vi "Teleop.vi"   [LabVIEW 2016]
doc: "This VI is called for each TeleOp packet received from the DS where the robot is not disabled. It is often used to read from the joysticks and update I/O or to update setpoints for timed control loops. It should complete and return within 20 milliseconds or it may miss DS packets."
uses:
  <vilib>/Rock Robotics/WPI/Utilities/WPI_GetSetVariantRefNum.vi
  External/2ndContollerStatus.vi
  External/External.lvlib
types:
  T1 = enum16{"A", "B", "X", "Y", "LB", "RB", "Back", "Start", "Left Joystick Pressure Button", "Right Joystick Pressure Button"}
  T2 = enum16{"Left X Axis", "Left Y Axis", "Left Trigger", "Right Trigger", "Right X Axis", "Right Y Axis"}
  T3 = enum16{"A", "B", "X", "Y", "LB", "RB", "Back", "Start"}
  T4 = typedef "WPI_JoystickDevRef.ctl" = cluster{"Device":T5}
  T5 = typedef "WPI_JoystickDeviceEnum.ctl" = enum16{"USB 0", "USB 1", "USB 2", "USB 3", "USB 4", "USB 5"}
  T6 = typedef "WPI_RobotDriveDevRef.ctl" = cluster{"DevStatus":errorcluster, "Motors[]":T7[], "Square Inputs":bool, "Max Output":dbl}
  T7 = typedef "WPI_MotorControlDeviceRef.ctl" = cluster{"DeviceStatus":errorcluster, "Type":T8, "PWM":cluster{"PWM Channel":T9, "DeadBand":T10}, "CAN":cluster{"Device Number":u8, "SetOutput VI Ref":variant, "GetOutput VI Ref":variant, "Enable VI Ref":variant, "Disable VI Ref":variant, "Data":variant}, "Invert":bool}
  T8 = typedef "WPI_MotorControlType.ctl" = enum16{"PWM", "CAN"}
  T9 = typedef "FPGA_DIOPWMChannel.ctl" = enum8{"PWM 0", "PWM 1", "PWM 2", "PWM 3", "PWM 4", "PWM 5", "PWM 6", "PWM 7", "PWM 8", "PWM 9", "PWM MXP 0", "PWM MXP 1", "PWM MXP 2", "PWM MXP 3", "PWM MXP 4", "PWM MXP 5", "PWM MXP 6", "PWM MXP 7", "PWM MXP 8", "PWM MXP 9", "Invalid"}
  T10 = typedef "WPI_PWMDeadband.ctl" = cluster{"Name":string, "maxPositivePwm":i32, "minPositivePwm":i32, "centerPwm":i32, "maxNegativePwm":i32, "minNegativePwm":i32, "angularRange":u16}
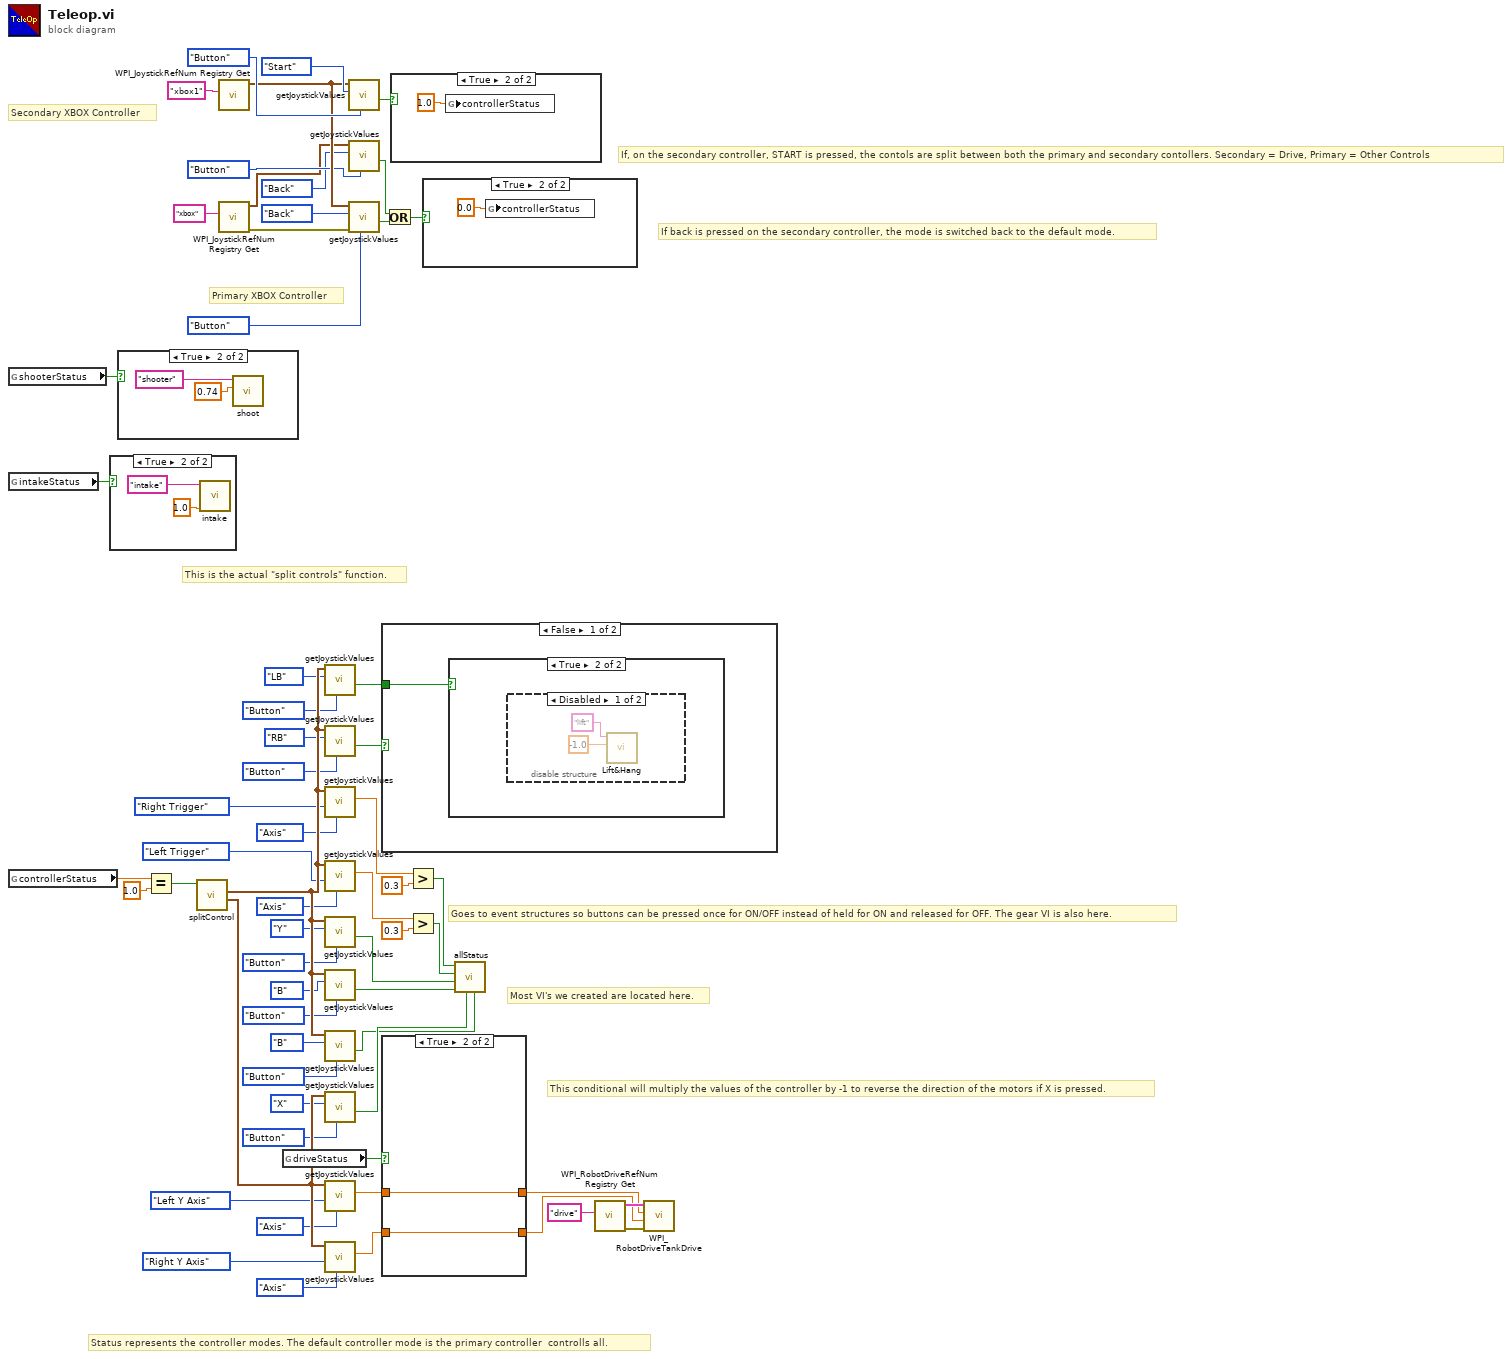
[diagram p0: block diagram]
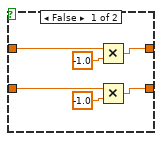
[diagram p2: hidden frame]
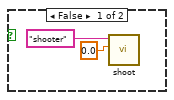
[diagram p3: hidden frame]
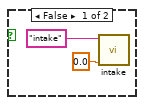
[diagram p4: hidden frame]
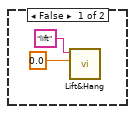
[diagram p5: hidden frame]
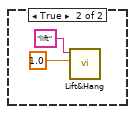
[diagram p7: hidden frame]
diagram:
  # "This is the actual \"split controls\" function."
  # "Most VI's we created are located here."
  # "This conditional will multiply the values of the controller by -1 to reverse the direction of the motors if X is pressed."
  # "Goes to event structures so buttons can be pressed once for ON/OFF instead of held for ON and released for OFF. The gear VI is also here."
  # "Status represents the controller modes. The default controller mode is the primary controller  controlls all."
  # "Secondary XBOX Controller"
  # "Primary XBOX Controller"
  # "If back is pressed on the secondary controller, the mode is switched back to the default mode."
  # "If, on the secondary controller, START is pressed, the contols are split between both the primary and secondary contollers. Secondary = Drive, Primary = Other Controls"
  n1 = global read "2ndContollerStatus.vi" "shooterStatus"() -> (w35:bool)
  n2 = global read "2ndContollerStatus.vi" "intakeStatus"() -> (w36:bool)
  n3 = global read "2ndContollerStatus.vi" "controllerStatus"() -> (w38:dbl)
  n4 = case shown="True" w36 {
    frame False {
      n5 = call "intake.vi"("intakeSpeed"=0.0, "intake"="intake") -> ()  [unwired: 9 in, 1 out]
    }
    frame True {
      n6 = call "intake.vi"("intakeSpeed"=1.0, "intake"="intake") -> ()  [unwired: 9 in, 1 out]
    }
  }
  n7 = case shown="True" w35 {
    frame False {
      n8 = call "shoot.vi"("Motor Power"=0.0, "refnum name"="shooter") -> ()  [unwired: 9 in, 1 out]
    }
    frame True {
      n9 = call "shoot.vi"("Motor Power"=0.74, "refnum name"="shooter") -> ()  [unwired: 9 in, 1 out]
    }
  }
  n10 = Equal?(x=w38, y=1.0) -> (x = y?=w24:bool)
  n11 = call "splitControl.vi"("driveStatus"=w24) -> ("JoystickDevRef 2"=w22:T4, "JoystickDevRef"=w23:T4)  [unwired: 9 in]
  n12 = call <vilib>:"WPI_JoystickRefNum Registry Get.vi"("refnum name"="xbox1" ("xbox1")) -> ("JoystickDevRef"=w57:T4)  [unwired: 9 in, 1 out]
  n13 = call <vilib>:"WPI_JoystickRefNum Registry Get.vi"("refnum name"="xbox" ("xbox")) -> ("error out"=w56:errorcluster, "JoystickDevRef"=w49:T4)  [unwired: 9 in]
  n14 = global read "2ndContollerStatus.vi" "driveStatus"() -> (w30:bool)
  n15 = call "getJoystickValues.vi"("Mode"=enum16{"Axis", "Button", "POV"}."Button", "buttonType"=T1."LB", "JoystickDevRef"=w23) -> ("Button Pressed"=w46:bool)  [unwired: 5 in, 3 out]
  n16 = call "getJoystickValues.vi"("Mode"=enum16{"Axis", "Button", "POV"}."Button", "buttonType"=T1."RB", "JoystickDevRef"=w23) -> ("Button Pressed"=w47:bool)  [unwired: 5 in, 3 out]
  n17 = call "getJoystickValues.vi"("Mode"=enum16{"Axis", "Button", "POV"}."Axis", "axisType"=T2."Right Trigger", "JoystickDevRef"=w23) -> ("Value"=w40:dbl)  [unwired: 5 in, 3 out]
  n18 = call "getJoystickValues.vi"("Mode"=enum16{"Axis", "Button", "POV"}."Axis", "axisType"=T2."Left Trigger", "JoystickDevRef"=w23) -> ("Value"=w39:dbl)  [unwired: 5 in, 3 out]
  n19 = call "getJoystickValues.vi"("Mode"=enum16{"Axis", "Button", "POV"}."Button", "buttonType"=T1."Y", "JoystickDevRef"=w23) -> ("Button Pressed"=w21:bool)  [unwired: 5 in, 3 out]
  n20 = call "getJoystickValues.vi"("Mode"=enum16{"Axis", "Button", "POV"}."Button", "buttonType"=T1."B", "JoystickDevRef"=w23) -> ("Button Pressed"=w27:bool)  [unwired: 5 in, 3 out]
  n21 = call "getJoystickValues.vi"("Mode"=enum16{"Axis", "Button", "POV"}."Button", "buttonType"=T1."B", "JoystickDevRef"=w23) -> ("Button Pressed"=w25:bool)  [unwired: 5 in, 3 out]
  n22 = call "getJoystickValues.vi"("Mode"=enum16{"Axis", "Button", "POV"}."Button", "buttonType"=T1."X", "JoystickDevRef"=w22) -> ("Button Pressed"=w26:bool)  [unwired: 5 in, 3 out]
  n23 = call "getJoystickValues.vi"("Mode"=enum16{"Axis", "Button", "POV"}."Axis", "axisType"=T2."Left Y Axis", "JoystickDevRef"=w22) -> ("Value"=w33:dbl)  [unwired: 5 in, 3 out]
  n24 = call "getJoystickValues.vi"("Mode"=enum16{"Axis", "Button", "POV"}."Axis", "axisType"=T2."Right Y Axis", "JoystickDevRef"=w22) -> ("Value"=w31:dbl)  [unwired: 5 in, 3 out]
  n25 = call "getJoystickValues.vi"("Mode"=enum16{"Axis", "Button"}."Button", "buttonType"=T3."Start", "JoystickDevRef"=w57) -> ("Button Pressed"=w52:bool)  [unwired: 5 in, 3 out]
  n26 = call "getJoystickValues.vi"("Mode"=enum16{"Axis", "Button"}."Button", "buttonType"=T3."Back", "JoystickDevRef"=w49) -> ("Button Pressed"=w50:bool)  [unwired: 5 in, 3 out]
  n27 = call "getJoystickValues.vi"("Mode"=enum16{"Axis", "Button"}."Button", "error in (no error)"=w56, "buttonType"=T3."Back", "JoystickDevRef"=w57) -> ("Button Pressed"=w51:bool)  [unwired: 4 in, 3 out]
  n28 = case shown="False" w47 {
    tunnel: w46 -> [w71 _]
    frame False {
      n29 = case shown="True" w71 {
        frame False {
          n30 = call "Lift&Hang.vi"("status"=0.0, "refnum name"="lift" ("lift")) -> ()  [unwired: 9 in, 1 out]
        }
        frame True {
          n31 = disable-structure shown="Disabled" {
            frame Disabled {
              n32 = call "Lift&Hang.vi"("status"=-1.0, "refnum name"="lift" ("lift")) -> ()  [unwired: 9 in, 1 out]
            }
            frame Enabled {
            }
          }
        }
      }
    }
    frame True {
      n33 = call "Lift&Hang.vi"("status"=1.0, "refnum name"="lift" ("lift")) -> ()  [unwired: 9 in, 1 out]
    }
  }
  n34 = case shown="True" w30 {
    tunnel: [w81 w85] -> w34
    tunnel: w33 -> [w83 w85]
    tunnel: [w79 w84] -> w32
    tunnel: w31 -> [w80 w84]
    frame False {
      n35 = Multiply(x=w83, y=-1.0) -> (x*y=w81:dbl)
      n36 = Multiply(x=w80, y=-1.0) -> (x*y=w79:dbl)
    }
    frame True {
    }
  }
  n37 = Or(x=w50, y=w51) -> (x .or. y?=w48:bool)
  n38 = case shown="True" w52 {
    frame False {
    }
    frame True {
      n39 = global write "2ndContollerStatus.vi" "controllerStatus"(1.0 ("status")) -> ()
    }
  }
  n40 = Greater?(x=w40, y=0.3) -> (0:w29:bool)
  n41 = Greater?(x=w39, y=0.3) -> (0:w28:bool)
  n42 = case shown="True" w48 {
    frame False {
    }
    frame True {
      n43 = global write "2ndContollerStatus.vi" "controllerStatus"(0.0 ("status")) -> ()
    }
  }
  n44 = call "allStatus.vi"("intake"=w25, "drive"=w26, "gear"=w27, "shooter"=w21, "hopper1"=w28, "hopper0"=w29) -> ()  [unwired: 6 in]
  n45 = call <vilib>:"WPI_RobotDriveRefNum Registry Get.vi"("refnum name"="drive") -> ("error out"=w44:errorcluster, "RobotDriveDevRef"=w45:T6)  [unwired: 9 in]
  n46 = call <vilib>:"WPI_RobotDriveTankDrive.vi"("error in (no error)"=w44, "Right axis value"=w32, "Left axis value"=w34, "RobotDriveDevRef"=w45) -> ()  [unwired: 5 in, 3 out]
